vi "Message - Confirm.vi"(8 "error in":errorcluster, 11 "Message In":string="Tittle") -> (0 "error out":errorcluster, 3 "Confirm":bool)   [LabVIEW 2014]
panel:
  out "Message Out":string="Tittle"
  in  "Confirm Button":bool
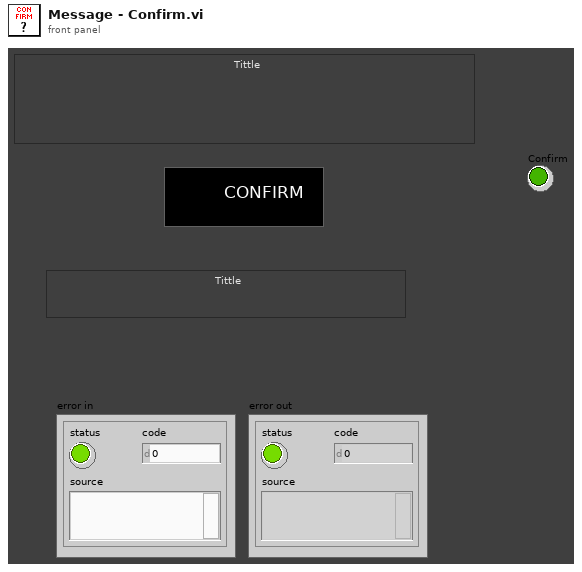
[diagram p1: front panel]
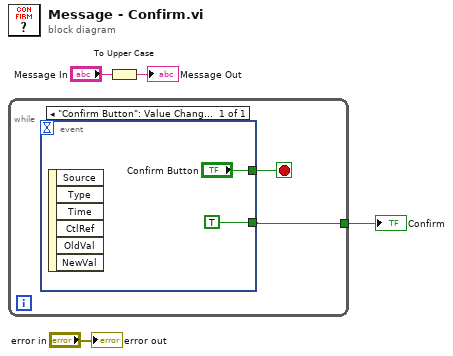
[diagram p0: block diagram]
diagram:
  n1 = while {
    tunnel: [w5] -> w1
    stop <- w6 stop-if-true
    n2 = event shown="[0] \"Confirm Button\": Value Change" {
      selector: _ -> [_]
      dyn-events: _ -> [_]
      timeout: _ -> [_]
      tunnel: ["Confirm Button"] -> w6
      tunnel: [TRUE] -> w5
      event "Confirm Button": Value Change {
        n3 = event-data() -> ()  [unwired: 1 in, 6 out]
      }
    }
  }
  "Confirm" <- w1
  n4 = To Upper Case(1:"Message In") -> (0:→"Message Out":string)
  "error out" <- "error in"
